vi "SolutionBuilder.vi"() -> ()   [LabVIEW 2020, in "SolutionBuilder.lvlib"]
uses:
  SolutionBuilder.lvlib
  Private/Options.ctl
panel:
  out "source":string
  out "code":i32
  out "status":bool
  out "Results":i32(listbox)
  in  "Preview?":bool
  in  "Path":path
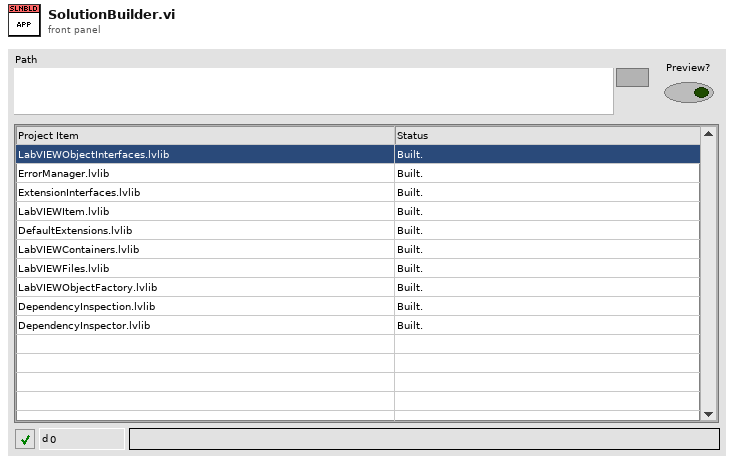
[diagram p1: front panel]
types:
  T1 = typedef "SolutionBuilder.lvlib/Options.ctl" = cluster{"Path":path, "Preview?":bool, "Quiet?":bool, "Show help?":bool}
  T2 = cluster{"UpdateList":refnum<user-event>, "ItemBuilt":refnum<user-event>, "Stop":refnum<user-event>}
  T3 = typedef "SolutionBuilder.lvlib/ItemInfo.ctl" = map{string, T4}
  T4 = typedef "SolutionBuilder.lvlib/ProjectInfo.ctl" = cluster{"Deps":set{string}, "FileInfo":T5}
  T5 = typedef "FileInfo.ctl" = cluster{"Library ref":refnum<vi>, "Target path":path, "Source name":string, "Build spec name":string}
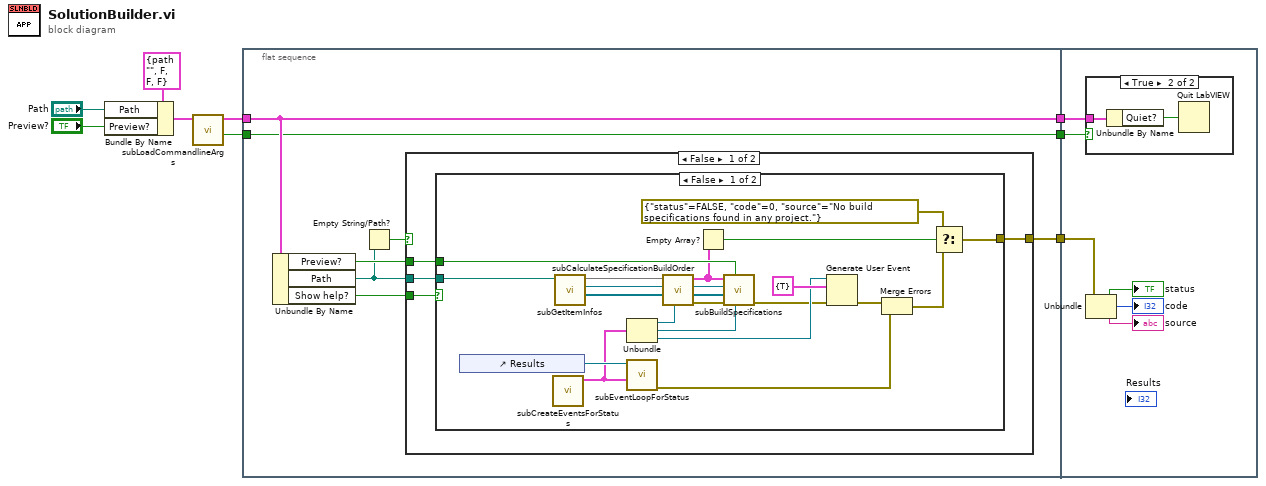
[diagram p0: block diagram]
diagram:
  n1 = Bundle By Name(cluster=T1 {"Path"=path "", "Preview?"=FALSE, "Quiet?"=FALSE, "Show help?"=FALSE} ("Options in"), "Path"="Path", "Preview?"="Preview?") -> (w4:T1)
  n2 = call "subLoadCommandlineArgs.vi"("Options in"=w4) -> ("From command line?"=w2:bool, "Options"=w8:T1)  [unwired: 9 in]
  n3 = flat-sequence {
    tunnel: [w16] -> w9
    tunnel: w8 -> [w16]
    tunnel: [w14] -> w3
    tunnel: w2 -> [w10]
    tunnel: [w10] -> w1
    tunnel: w9 -> [w46]
    tunnel: w3 -> [w42]
    tunnel: w1 -> [w41]
    frame #0 {
      n4 = Unbundle By Name(w16) -> ("Preview?"=w15:bool, "Path"=w12:path, "Show help?"=w13:bool)
      n5 = Empty String/Path?(string/path=w12) -> (empty?=w11:bool)
      n6 = case shown="False" w11 {
        tunnel: w15 -> [w20 _]
        tunnel: w12 -> [w19 _]
        tunnel: [w18 _] -> w14
        tunnel: w13 -> [w17 _]
        frame False {
          n7 = case shown="False" w17 {
            tunnel: w20 -> [w29 _]
            tunnel: w19 -> [w28 _]
            tunnel: [w23 _] -> w18
            frame False {
              n8 = control-ref of="Results"() -> (w39:refnum<vi>)
              n9 = call "subCreateEventsForStatus.vi"() -> ("Events"=w38:T2)  [unwired: 11 in]
              n10 = call "subGetItemInfos.vi"("Path"=w28) -> ("Project refs"=w21:refnum<vi>[], "Local Host App Instance"=w22:refnum<vi>, "Item info"=w40:T3)  [unwired: 8 in]
              n11 = Unbundle(w38) -> ("UpdateList"=w37:refnum<user-event>, "ItemBuilt"=w33:refnum<user-event>, "Stop"=w34:refnum<user-event>)
              n12 = call "subEventLoopForStatus.vi"("Events"=w38, "MulticolumnListbox in"=w39) -> ("error out"=w35:errorcluster)  [unwired: 9 in]
              n13 = call "subCalculateSpecificationBuildOrder.vi"("UpdateList"=w37, "Item info"=w40) -> ("error out"=w32:errorcluster, "Dependency order"=w27:T5[])  [unwired: 8 in]
              n14 = Empty Array?(array=w27) -> (empty?=w26:bool)
              n15 = call "subBuildSpecifications.vi"("ItemBuilt"=w33, "Preview?"=w29, "error in (no error)"=w32, "Project refs"=w21, "Local Host App Instance"=w22, "Dependency order"=w27) -> ("error out"=w31:errorcluster)  [unwired: 5 in]
              n16 = Generate User Event(user event=w34, event data cluster=cluster{"Stop":bool} {"Stop"=TRUE} ("event data"), error in=w31) -> (error out=w30:errorcluster)  [unwired: 1 in, 1 out]
              n17 = Merge Errors(w30, w35) -> (w25:errorcluster)
              n18 = Select(t=errorcluster {"status"=FALSE, "code"=0, "source"="No build specifications found in any project."}, s=w26, f=w25) -> (s? t:f=w23:errorcluster)
            }
            frame True {
            }
          }
        }
        frame True {
        }
      }
    }
    frame #1 {
      n19 = case shown="True" w41 {
        tunnel: w46 -> [_ w48]
        frame False {
        }
        frame True {
          n20 = Unbundle By Name(w48) -> ("Quiet?"=w47:bool)
          n21 = Quit LabVIEW(quit? (T)=w47) -> ()
        }
      }
      n22 = Unbundle(w42) -> ("status"=→"status":bool, "code"=→"code":i32, "source"=→"source":string)
    }
  }
